vi "Select.vi"(8 "error in (no error)":errorcluster caption="entrée d'erreur (pas d'erreur)", 11 "Database Drivers en entrée":refnum<class "Database Drivers.lvclass">) -> (0 "error out":errorcluster caption="sortie d'erreur", 3 "Database Drivers en sortie":refnum<class "Database Drivers.lvclass">)   [LabVIEW 2020, in "Library Instrument & Equipement.lvlib" / "Library Database.lvlib" / "Database Drivers.lvclass"]
uses:
  Database Drivers.lvclass
  Database Drivers.lvclass/Database Drivers.ctl
  <vilib>/addons/database/NI_Database_API.lvlib
  <vilib>/addons/database/Recordset.llb/Rec Get Recordset Properties (R).vi
  <vilib>/addons/database/Recordset.llb/Rec Fetch Recordset Data (R).vi
  <vilib>/addons/database/Connection.llb/Conn Execute.vi
  <vilib>/addons/database/Auxilliary.llb/DB Tools Cursor Type.ctl
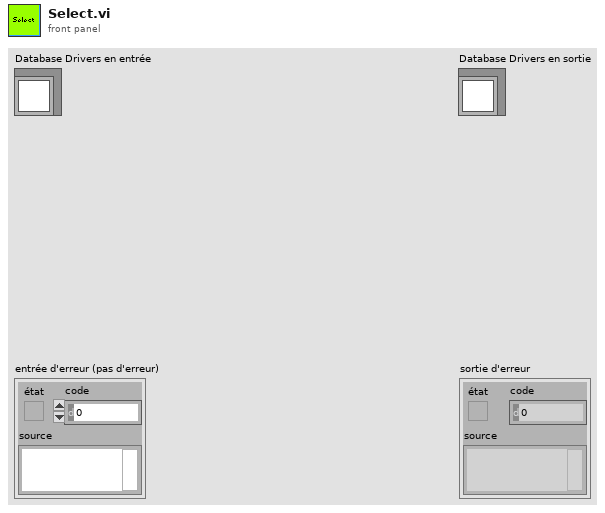
[diagram p1: front panel]
types:
  T1 = typedef "NI_Database_API.lvlib/DB Tools Cursor Type.ctl" = enum16{"forward-only", "keyset", "dynamic", "static"}
  T2 = typedef "NI_Database_API.lvlib/Conn ObjectReference.ctl" = refnum<k1>
  T3 = typedef "NI_Database_API.lvlib/Rec ObjectReference.ctl" = refnum<k1>
  T4 = typedef "NI_Database_API.lvlib/Rec Properties.ctl" = cluster{"column count":i32, "record index":i32, "record count":i32, "bof?":bool, "eof?":bool, "cursor type":T1, "cache size":i32, "state":enum16{"closed", "open"}}
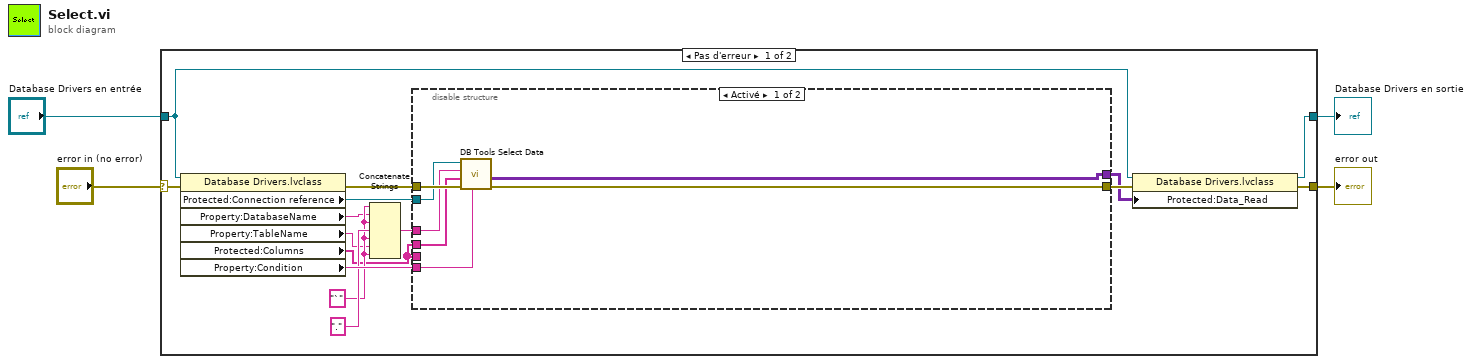
[diagram p0: block diagram]
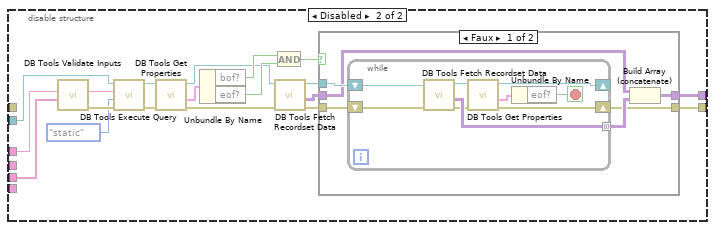
[diagram p2: hidden frame]
diagram:
  n1 = case shown="Pas d'erreur" "error in (no error)" {
    selector: "error in (no error)" -> [w19 w64]
    tunnel: [w16 w64] -> w3
    tunnel: [w17 w63] -> w1
    tunnel: "Database Drivers en entrée" -> [w18 w63]
    frame No Error {
      w9 = "`" ("chaîne")
      n2 = property class="Database Drivers.lvclass"(reference=w18, error in=w19) -> (error out=w15:errorcluster, "Protected:Connection reference"=w13:T2, "Property:DatabaseName"=w8:string, "Property:TableName"=w7:string, "Protected:Columns"=w5:string[], "Property:Condition"=w12:string)  [unwired: 1 out]
      n3 = Concatenate Strings(w9, w8, w9, "." ("chaîne"), w9, w7, w9) -> (w6:string)
      n4 = disable-structure shown="Activé" {
        disable-tunnel: w15 -> [w26 _]
        disable-tunnel: [w25 w28] -> w14
        disable-tunnel: w13 -> [w24 w45]
        disable-tunnel: w12 -> [w23 _]
        disable-tunnel: [w22 w29] -> w11
        disable-tunnel: w6 -> [w21 w43]
        disable-tunnel: w5 -> [w20 _]
        disable-tunnel: w5 -> [_ w44]
        frame Enabled {
          n5 = call <vilib>:"DB Tools Select Data.vi"("condition"=w23, "error in (no error)"=w26, "columns"=w20, "table"=w21, "connection reference"=w24) -> ("error out"=w25:errorcluster, "data"=w22:variant[][])  [unwired: 1 in, 1 out]
        }
        frame Disabled {
          n6 = call <vilib>:"DB Tools Validate Inputs.vi"("columns"=w44, "table"=w43) -> ("error out"=w42:errorcluster, "table out"=w41:string)  [unwired: 3 in, 1 out]
          n7 = call-poly <vilib>:"DB Tools Execute Query.vi"("error in (no error)"=w42, "cursor type"=DB_Tools_Cursor_Type."static", "SQL query"=w41, "connection reference"=w45) -> ("error out"=w40:errorcluster, "recordset reference"=w39:T3)  [unwired: 4 in]
          n8 = call-poly <vilib>:"DB Tools Get Properties.vi"("error in (no error)"=w40, "recordset reference"=w39) -> ("error out"=w33:errorcluster, "recordset properties"=w38:T4, "recordset reference out"=w31:T3)  [unwired: 3 in]
          n9 = Unbundle By Name(w38) -> ("bof?"=w37:bool, "eof?"=w36:bool)
          n10 = And(x=w37, y=w36) -> (x .and. y?=w35:bool)
          n11 = call-poly <vilib>:"DB Tools Fetch Recordset Data.vi"("error in (no error)"=w33, "recordset reference"=w31) -> ("error out"=w32:errorcluster, "recordset data"=w30:variant[][], "recordset reference out"=w34:T3)  [unwired: 3 in]
          n12 = case shown="Faux" w35 {
            tunnel: w34 -> [w51 _]
            tunnel: w32 -> [w50 w61]
            tunnel: w30 -> [w48 w62]
            tunnel: [w47 w62] -> w29
            tunnel: [w46 w61] -> w28
            frame False {
              n13 = while {
                shift-right: [w55] -> w46
                shift-left: w50 -> [w52]
                tunnel: [w59] -> w49 mode=concatenating
                shift-right: [w56] -> _
                shift-left: w51 -> [w53]
                stop <- w58 stop-if-true
                n14 = call-poly <vilib>:"DB Tools Fetch Recordset Data.vi"("error in (no error)"=w52, "recordset reference"=w53) -> ("error out"=w54:errorcluster, "recordset data"=w59:variant[][], "recordset reference out"=w57:T3)  [unwired: 3 in]
                n15 = call-poly <vilib>:"DB Tools Get Properties.vi"("error in (no error)"=w54, "recordset reference"=w57) -> ("error out"=w55:errorcluster, "recordset properties"=w60:T4, "recordset reference out"=w56:T3)  [unwired: 3 in]
                n16 = Unbundle By Name(w60) -> ("eof?"=w58:bool)
              }
              n17 = Build Array (concatenate)(w48, w49) -> (w47:variant[][])
            }
            frame True {
            }
          }
        }
      }
      n18 = property class="Database Drivers.lvclass"(reference=w18, error in=w14, "Protected:Data_Read"=w11) -> (reference out=w17:refnum<class "Database Drivers.lvclass">, error out=w16:errorcluster)
    }
    frame Error {
    }
  }
  "error out" <- w3
  "Database Drivers en sortie" <- w1
